vi "target_gm.vi"   [LabVIEW 2011]
uses:
  Input - Cluster gas.ctl
  Output - Cluster gas.ctl
  <vilib>/Platform/TimedLoop/XDataNode/timing_clust.ctl
  <vilib>/Platform/TimedLoop/XDataNode/nitl_modes.ctl
  <vilib>/Platform/TimedLoop/XDataNode/wakeup.ctl
  <vilib>/Platform/TimedLoop/XDataNode/XDataNode.xnode
  <vilib>/Platform/TimedLoop/XDataNode/XDNodeRunTimeDep.lvlib
panel:
  # "The Network Variable Engine and Variable Client Support must be installed on the RT target\nfor this application to function properly. If the Network Variable Engine is not supported on\nthe target (e.g.  FP-2000 with <32MB of RAM), open the project and move the variable library\nto My Computer in the project. Doing this will deploy the variables to localhost but\nwill still require that Variable Client Support be installed on the RT target."
types:
  T1 = typedef "XDNodeRunTimeDep.lvlib/timing_clust.ctl" = cluster{"Expected End [f-1]":u64, "Actual End [f-1]":u64, "Finished Late? [f-1]":bool, "Expected End [i-1]":u64, "Actual End [i-1]":u64, "Finished Late? [i-1]":bool, "Expected Start [i]":u64, "Actual Start [i]":u64, "Expected Start [f]":u64, "Actual Start [f]":u64, "Source Name":string, "Structure Name":string, "Period":i64, "Deadline":i64, "Offset":i64, "Start":i64, "Priority":i32, "Timeout":i32, "Mode":T2, "Wakeup Reason":T3, "Error":errorcluster, "Source Type":string, "Secondary Source Type":string, "Global End Time":u64, "Global Start Time":u64, "Frame Duration":u64, "Iteration Duration":u64, "Assigned CPU":i32, "I/O Scan Engine Mode":u32}
  T2 = typedef "XDNodeRunTimeDep.lvlib/nitl_modes.ctl" = enum32{"No Change", "Process missed periods, maintain original phase", "Discard missed periods, maintain original phase", "Process missed periods, ignore original phase", "Discard missed periods, ignore original phase"}
  T3 = typedef "XDNodeRunTimeDep.lvlib/wakeup.ctl" = enum32{"Normal", "Aborted", "Asynchronous wakeup", "Timing source error", "Timed loop error", "Timeout"}
  T4 = cluster{"STOP":bool, "sqlite_file":string, "gas_values.timestamp":timestamp, "db_write":i64, "output cluster timestamp":timestamp}
  T5 = typedef "Input - Cluster gas.ctl" = cluster{"GM P-1":bool, "GM P-2":bool, "measuring point":u32, "measuring mode":u8, "GM-V1,2":bool, "GM-V3,4":bool, "GM-V5":bool, "measuring volume":u32}
  T6 = typedef "Output - Cluster gas.ctl" = cluster{"B2G2 MR V1.1 AUF":bool, "B2G2 MR V1.1 ZU":bool, "B2G2 MR V1 AUF":bool, "B2G2 MR V1 ZU":bool, "B2G1 T2 V1 AUF":bool, "B2G1 T2 V1 ZU":bool, "B2G1 T2 V1.1 AUF":bool, "B2G1 T2 V1.1 ZU":bool, "B2G2 T2 V1 AUF":bool, "B2G2 T2 V1 ZU":bool, "B2G2 T2 V1.1 ZU":bool, "B2G2 T2 V1.1 AUF":bool, "B2G1 MR V1 AUF":bool, "B2G1 MR V1 ZU":bool, "B2G1 MR V1.1 AUF":bool, "B2G1 MR V1.1 ZU":bool, "B2G1 HR V1 AUF":bool, "B2G1 HR V1 ZU":bool, "B2G1 HR V1.1 AUF":bool, "B2G1 HR V1.1 ZU":bool, "Fab1 HR V1 AUF":bool, "Fab1 HR V1 ZU":bool, "Fab1 HR V1.1 AUF":bool, "Fab1 HR V1.1 ZU":bool, "Fab1 MR V1 AUF":bool, "Fab1 MR V1 ZU":bool, "Fab1 MR V1.1 AUF":bool, "Fab1 MR V1.1 ZU":bool, "Fab1 BL V1 AUF":bool, "Fab1 BL V1 ZU":bool, "Fab1 BL V1.1 AUF":bool, "Fab1 BL V1.1 ZU":bool, "Fab2 HR V1 AUF":bool, "Fab2 HR V1 ZU":bool, "Fab2 HR V1.1 AUF":bool, "Fab2 HR V1.1 ZU":bool, "Fab2 MR V1 AUF":bool, "Fab2 MR V1 ZU":bool, "Fab2 MR V1.1 AUF":bool, "Fab2 MR V1.1 ZU":bool, "GA1 ch4 [%]":dbl, "GA1 co2 [%]":dbl, "GA1 h2 [%]":dbl, "GM P1 RUN":bool, "GM V-1 AUF":bool, "GM V-1 ZU":bool, "GM V-2 AUF":bool, "GM V-2 ZU":bool, "GM V-3 AUF":bool, "GM V-3 ZU":bool, "GM V-4 AUF":bool, "GM V-4 ZU":bool, "GM P2 RUN":bool, "GM GZ-1 [imp]":u32, "GM DS-2 [bar]":dbl, "GM DS-1 [bar]":dbl, "GM TS-1 [°C]":dbl, "GM TS-2[°C]":dbl, "gas_values":cluster{"timestamp":timestamp, "GM DS-2 [bar]":dbl, "GA1 ch4 [%]":dbl, "GA1 co2 [%]":dbl, "GA1 h2 [%]":dbl, "GM DS-1 [bar]":dbl, "GM TS-1 [°C]":dbl, "GM TS-2 [°C]":dbl, "GM GZ-1 [l]":dbl, "empty":bool, "measuring point":u8}, "measuring mode":u8}
  T7 = cluster{"STOP":bool, "measuring point":u32, "measuring mode t-1":u8, "measuring mode t-2":u8, "measuring volume":u32, "gas_values":cluster{"GA1 ch4 [%]":dbl, "GA1 co2 [%]":dbl, "GA1 h2 [%]":dbl, "empty":bool, "measuring point":u8}}
  T8 = cluster{"GA1 ch4 [%]":dbl, "GA1 co2 [%]":dbl, "GA1 h2 [%]":dbl, "empty":bool, "measuring point":u8}
  T9 = cluster{"timestamp":timestamp, "GM DS-2 [bar]":dbl, "GA1 ch4 [%]":dbl, "GA1 co2 [%]":dbl, "GA1 h2 [%]":dbl, "GM DS-1 [bar]":dbl, "GM TS-1 [°C]":dbl, "GM TS-2 [°C]":dbl, "GM GZ-1 [l]":dbl, "empty":bool, "measuring point":u8}
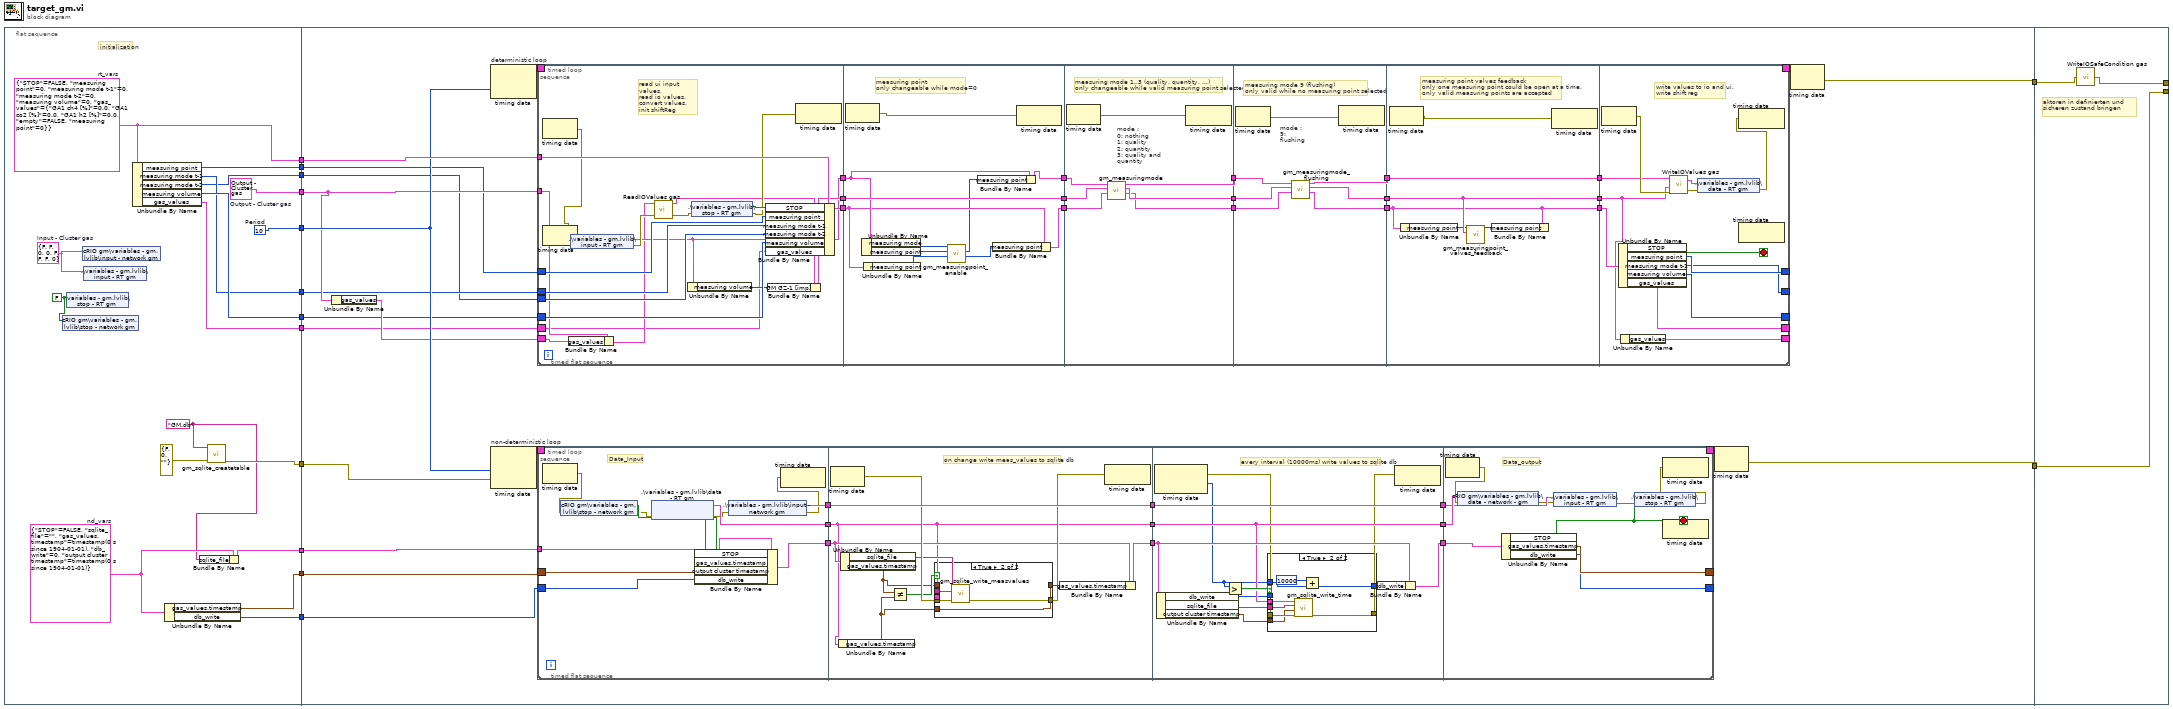
[diagram p0: block diagram]
diagram:
  n1 = flat-sequence {
    tunnel: [w20] -> w14
    tunnel: [w31] -> w13
    tunnel: [w30] -> w12
    tunnel: [w22] -> w9
    tunnel: [w19] -> w8
    tunnel: [w27] -> w7
    tunnel: [w23] -> w6
    tunnel: [w24] -> w5
    tunnel: [w18] -> w4
    tunnel: [w17] -> w3
    tunnel: [w16] -> w2
    tunnel: [w15] -> w1
    tunnel: w14 -> [w46]
    tunnel: w13 -> [w45]
    tunnel: w12 -> [w41]
    tunnel: [w44] -> w11
    tunnel: [w43] -> w10
    tunnel: w9 -> [w42]
    tunnel: w8 -> [w39]
    tunnel: w7 -> [w38]
    tunnel: w6 -> [w37]
    tunnel: w5 -> [w36]
    tunnel: w4 -> [w35]
    tunnel: w3 -> [w34]
    tunnel: w2 -> [w33]
    tunnel: w1 -> [w32]
    tunnel: w11 -> [w304]
    tunnel: w10 -> [w302]
    tunnel: [w303] -> _
    tunnel: [w304] -> _
    frame #0 {
      w26 = FALSE ("stop - RT gas")
      w21 = "GM.db" ("Database File")
      w25 = T4 {"STOP"=FALSE, "sqlite_file"="", "gas_values.timestamp"=timestamp(0 s since 1904-01-01), "db_write"=0, "output cluster timestamp"=timestamp(0 s since 1904-01-01)}  # nd_vars
      w29 = T5 {"GM P-1"=FALSE, "GM P-2"=FALSE, "measuring point"=0, "measuring mode"=0, "GM-V1,2"=FALSE, "GM-V3,4"=FALSE, "GM-V5"=FALSE, "measuring volume"=0}  # Input - Cluster gas
      w30 = T6 {"B2G2 MR V1.1 AUF"=FALSE, "B2G2 MR V1.1 ZU"=FALSE, "B2G2 MR V1 AUF"=FALSE, "B2G2 MR V1 ZU"=FALSE, "B2G1 T2 V1 AUF"=FALSE, "B2G1 T2 V1 ZU"=FALSE, "B2G1 T2 V1.1 AUF"=FALSE, "B2G1 T2 V1.1 ZU"=FALSE, "B2G2 T2 V1 AUF"=FALSE, "B2G2 T2 V1 ZU"=FALSE, "B2G2 T2 V1.1 ZU"=FALSE, "B2G2 T2 V1.1 AUF"=FALSE, "B2G1 MR V1 AUF"=FALSE, "B2G1 MR V1 ZU"=FALSE, "B2G1 MR V1.1 AUF"=FALSE, "B2G1 MR V1.1 ZU"=FALSE, "B2G1 HR V1 AUF"=FALSE, "B2G1 HR V1 ZU"=FALSE, "B2G1 HR V1.1 AUF"=FALSE, "B2G1 HR V1.1 ZU"=FALSE, "Fab1 HR V1 AUF"=FALSE, "Fab1 HR V1 ZU"=FALSE, "Fab1 HR V1.1 AUF"=FALSE, "Fab1 HR V1.1 ZU"=FALSE, "Fab1 MR V1 AUF"=FALSE, "Fab1 MR V1 ZU"=FALSE, "Fab1 MR V1.1 AUF"=FALSE, "Fab1 MR V1.1 ZU"=FALSE, "Fab1 BL V1 AUF"=FALSE, "Fab1 BL V1 ZU"=FALSE, "Fab1 BL V1.1 AUF"=FALSE, "Fab1 BL V1.1 ZU"=FALSE, "Fab2 HR V1 AUF"=FALSE, "Fab2 HR V1 ZU"=FALSE, "Fab2 HR V1.1 AUF"=FALSE, "Fab2 HR V1.1 ZU"=FALSE, "Fab2 MR V1 AUF"=FALSE, "Fab2 MR V1 ZU"=FALSE, "Fab2 MR V1.1 AUF"=FALSE, "Fab2 MR V1.1 ZU"=FALSE, "GA1 ch4 [%]"=0.0, "GA1 co2 [%]"=0.0, "GA1 h2 [%]"=0.0, "GM P1 RUN"=FALSE, "GM V-1 AUF"=FALSE, "GM V-1 ZU"=FALSE, "GM V-2 AUF"=FALSE, "GM V-2 ZU"=FALSE, "GM V-3 AUF"=FALSE, "GM V-3 ZU"=FALSE, "GM V-4 AUF"=FALSE, "GM V-4 ZU"=FALSE, "GM P2 RUN"=FALSE, "GM GZ-1 [imp]"=0, "GM DS-2 [bar]"=0.0, "GM DS-1 [bar]"=0.0, "GM TS-1 [°C]"=0.0, "GM TS-2[°C]"=0.0, "gas_values"={"timestamp"=timestamp(0 s since 1904-01-01), "GM DS-2 [bar]"=0.0, "GA1 ch4 [%]"=0.0, "GA1 co2 [%]"=0.0, "GA1 h2 [%]"=0.0, "GM DS-1 [bar]"=0.0, "GM TS-1 [°C]"=0.0, "GM TS-2 [°C]"=0.0, "GM GZ-1 [l]"=0.0, "empty"=FALSE, "measuring point"=0}, "measuring mode"=0}  # Output - Cluster gas
      w20 = T7 {"STOP"=FALSE, "measuring point"=0, "measuring mode t-1"=0, "measuring mode t-2"=0, "measuring volume"=0, "gas_values"={"GA1 ch4 [%]"=0.0, "GA1 co2 [%]"=0.0, "GA1 h2 [%]"=0.0, "empty"=FALSE, "measuring point"=0}}  # rt_vars
      w31 = i64 10  # Period
      # "initialization"
      n2 = shared-variable "cRIO gm\\variables - gm.lvlib\\stop - network gm"(w26) -> ()  [unwired: 1 in, 1 out]
      n3 = shared-variable ".\\variables - gm.lvlib\\stop - RT gm"(w26) -> ()  [unwired: 1 in, 1 out]
      n4 = shared-variable "cRIO gm\\variables - gm.lvlib\\input - network gm"(w29) -> ()  [unwired: 1 in, 1 out]
      n5 = shared-variable ".\\variables - gm.lvlib\\input - RT gm"(w29) -> ()  [unwired: 1 in, 1 out]
      n6 = Unbundle By Name(w20) -> ("measuring point"=w18:u32, "measuring mode t-1"=w16:u8, "measuring mode t-2"=w15:u8, "measuring volume"=w17:u32, "gas_values"=w19:T8)
      n7 = Unbundle By Name(w25) -> ("gas_values.timestamp"=w23:timestamp, "db_write"=w24:i64)
      n8 = Bundle By Name(cluster=w25, "sqlite_file"=w21) -> (w22:T4)
      n9 = call "gm_sqlite_createtable.vi"("error in (no error)"=errorcluster {"status"=FALSE, "code"=0, "source"=""}, "Database File"=w21) -> ("error out"=w27:errorcluster)  [unwired: 9 in]
    }
    frame #1 {
      n10 = Unbundle By Name(w41) -> ("gas_values"=w40:T9)
      n11 = node-c288 ("Input Node")(w45) -> (w50:T1)  [unwired: 1 in]
      n12 = node-c288 ("Input Node")(w45, w38) -> (w48:T1)  [unwired: 1 in]
      n13 = timed-loop "deterministic loop" {
        timing: w50 -> [_]
        timing-out: [_] -> w49
        tunnel: w46 -> [w173]
        tunnel: w41 -> [w172]
        shift-right: [w171] -> _
        shift-left: w35 -> [w170]
        shift-right: [w169] -> _
        shift-left: w33 -> [w168]
        shift-left: w32 -> [w167]
        shift-right: [w166] -> _
        shift-left: w34 -> [w165]
        shift-right: [w164] -> _
        shift-left: w40 -> [w163]
        shift-right: [w162] -> _
        shift-left: w39 -> [w161]
        stop <- w286 stop-if-true
        n14 = timed-sequence {
          timing: _ -> [_]
          timing-out: _ -> [_]
          tunnel: w173 -> [w201]
          tunnel: w172 -> [w200]
          tunnel: [w193] -> w171
          tunnel: w170 -> [w192]
          tunnel: [w188] -> w169
          tunnel: w168 -> [w187]
          tunnel: w167 -> [w186]
          tunnel: [w185] -> w166
          tunnel: w165 -> [w184]
          tunnel: [w183] -> w164
          tunnel: w163 -> [w182]
          tunnel: [w181] -> w162
          tunnel: w161 -> [w180]
          n15 = timed-flat-sequence {
            tunnel: w201 -> [w220]
            tunnel: w200 -> [w205]
            tunnel: [w207] -> w199
            tunnel: [w216] -> w198
            tunnel: [w208] -> w197
            tunnel: w192 -> [w212]
            tunnel: w187 -> [w211]
            tunnel: w186 -> [w210]
            tunnel: w184 -> [w209]
            tunnel: w182 -> [w203]
            tunnel: w180 -> [w202]
            tunnel: w199 -> [w234]
            tunnel: [w227] -> w191
            tunnel: w198 -> [w231]
            tunnel: [w229] -> w190
            tunnel: w197 -> [w236]
            tunnel: [w236] -> w189
            tunnel: w191 -> [w243]
            tunnel: [w242] -> w179
            tunnel: w190 -> [w245]
            tunnel: [w244] -> w177
            tunnel: w189 -> [w247]
            tunnel: [w246] -> w175
            tunnel: w179 -> [w259]
            tunnel: [w258] -> w178
            tunnel: w177 -> [w255]
            tunnel: [w254] -> w176
            tunnel: w175 -> [w257]
            tunnel: [w256] -> w174
            tunnel: w178 -> [w271]
            tunnel: [w271] -> w196
            tunnel: w176 -> [w266]
            tunnel: [w266] -> w195
            tunnel: w174 -> [w269]
            tunnel: [w269] -> w194
            tunnel: w196 -> [w283]
            tunnel: w195 -> [w287]
            tunnel: w194 -> [w279]
            tunnel: [w282] -> w193
            tunnel: [w281] -> w188
            tunnel: [w280] -> w185
            tunnel: [w278] -> w183
            tunnel: [w277] -> w181
            frame #0 {
              # "read ui input values,\nread io values,\nconvert values,\ninit shiftReg"
              n16 = node-c288 ("Output Node")() -> (w214:errorcluster)  [unwired: 1 in]
              n17 = Bundle By Name(cluster=w205, "gas_values"=w203) -> (w204:T6)
              n18 = shared-variable ".\\variables - gm.lvlib\\input - RT gm"(error in=w214) -> (w207:T5, error out=w213:errorcluster)
              n19 = call "ReadIOValues gas.vi"("error in"=w213, "Output - Cluster gas"=w204) -> ("error out"=w217:errorcluster, "Output - Cluster gas"=w215:T6)  [unwired: 2 in]
              n20 = Unbundle By Name(w207) -> ("measuring volume"=w206:u32)
              n21 = shared-variable ".\\variables - gm.lvlib\\stop - RT gm"(error in=w217) -> (w219:bool, error out=w218:errorcluster)
              n22 = Bundle By Name(cluster=w220, "STOP"=w219, "measuring point"=w212, "measuring mode t-1"=w211, "measuring mode t-2"=w210, "measuring volume"=w209, "gas_values"=w202) -> (w216:T7)
              n23 = Bundle By Name(cluster=w215, "GM GZ-1 [imp]"=w206) -> (w208:T6)
              n24 = node-c288 ("Input Node")(w218) -> ()  [unwired: 1 out]
            }
            frame #1 {
              # "measuring point\nonly changeable while mode=0"
              n25 = node-c288() -> (w235:errorcluster)  [unwired: 1 in]
              n26 = Unbundle By Name(w234) -> ("measuring mode"=w233:u8, "measuring point"=w232:u32)
              n27 = Unbundle By Name(w231) -> ("measuring point"=w230:u32)
              n28 = call "gm_measuringpoint_enable.vi"("shift reg"=w230, "measuring point"=w232, "measuring mode"=w233) -> ("shift reg out"=w228:u32, "measuring point"=w226:u32)  [unwired: 6 in]
              n29 = Bundle By Name(cluster=w234, "measuring point"=w226) -> (w227:T5)
              n30 = Bundle By Name(cluster=w231, "measuring point"=w228) -> (w229:T7)
              n31 = node-c288(w235) -> ()  [unwired: 1 out]
            }
            frame #2 {
              # "measuring mode 1..3 (quality, quantity, ...)\nonly changeable while valid measuring point selected"
              # "mode :\n0: nothing\n1: quality\n2: quantity\n3: quality and quantity"
              n32 = node-c288() -> (w248:errorcluster)  [unwired: 1 in]
              n33 = call "gm_measuringmode.vi"("rt_vars in"=w245, "Output - Cluster gas in"=w247, "Input - Cluster gas in"=w243) -> ("rt_vars out"=w244:T7, "Output - Cluster gas out"=w246:T6, "Input - Cluster gas out"=w242:T5)  [unwired: 6 in]
              n34 = node-c288(w248) -> ()  [unwired: 1 out]
            }
            frame #3 {
              # "mode :\n9: flushing"
              # "measuring mode 9 (flushing)\nonly valid while no measuring point selected"
              n35 = node-c288() -> (w260:errorcluster)  [unwired: 1 in]
              n36 = call "gm_measuringmode_flushing.vi"("rt_vars in"=w255, "Output - Cluster gas in"=w257, "Input - Cluster gas in"=w259) -> ("rt_vars out"=w254:T7, "Output - Cluster gas out"=w256:T6, "Input - Cluster gas out"=w258:T5)  [unwired: 6 in]
              n37 = node-c288(w260) -> ()  [unwired: 1 out]
            }
            frame #4 {
              # "measuring point valves feedback \nonly one measuring point could be open at a time,\nonly valid measuring points are accepted"
              n38 = node-c288() -> (w270:errorcluster)  [unwired: 1 in]
              n39 = Unbundle By Name(w266) -> ("measuring point"=w268:u32)
              n40 = call "gm_measuringpoint_valves_feedback.vi"("Output - Cluster gas"=w269, "measuring point"=w268) -> ("measuring point"=w267:u32)  [unwired: 9 in]
              n41 = Bundle By Name(cluster=w266, "measuring point"=w267) -> ()  [unwired: 1 out]
              n42 = node-c288(w270) -> ()  [unwired: 1 out]
            }
            frame #5 {
              # "write values to io and ui,\nwrite shift reg"
              n43 = node-c288() -> (w285:errorcluster)  [unwired: 1 in]
              n44 = Unbundle By Name(w287) -> ("STOP"=w286:bool, "measuring point"=w282:u32, "measuring mode t-1"=w281:u8, "measuring volume"=w280:u32, "gas_values"=w277:T8)
              n45 = Unbundle By Name(w279) -> ("gas_values"=w278:T9)
              n46 = call "WriteIOValues gas.vi"("error in"=w285, "Output - Cluster gas"=w279, "input cluster"=w283) -> ("error out"=w284:errorcluster, "Output - Cluster gas 2"=w289:T6)  [unwired: 1 in]
              n47 = shared-variable ".\\variables - gm.lvlib\\data - RT gm"(w289, error in=w284) -> (error out=w288:errorcluster)
              n48 = node-c288(w288) -> ()  [unwired: 1 out]
            }
          }
        }
        n49 = node-c288() -> ()  [unwired: 1 in, 1 out]
        n50 = node-c288() -> ()  [unwired: 1 in, 1 out]
      }
      n51 = timed-loop "non-deterministic loop" {
        timing: w48 -> [_]
        timing-out: [_] -> w47
        tunnel: w42 -> [w55]
        shift-right: [w54] -> _
        shift-left: w37 -> [w53]
        shift-right: [w52] -> _
        shift-left: w36 -> [w51]
        stop <- w144 stop-if-true
        n52 = timed-sequence {
          timing: _ -> [_]
          timing-out: _ -> [_]
          tunnel: w55 -> [w69]
          tunnel: [w68] -> w54
          tunnel: w53 -> [w67]
          tunnel: [w60] -> w52
          tunnel: w51 -> [w56]
          n53 = timed-flat-sequence {
            tunnel: [w78] -> w58
            tunnel: [w79] -> w59
            tunnel: w69 -> [w81]
            tunnel: [w80] -> w57
            tunnel: w67 -> [w72]
            tunnel: w56 -> [w70]
            tunnel: w59 -> [w97]
            tunnel: [w97] -> w66
            tunnel: w58 -> [w92]
            tunnel: [w92] -> w64
            tunnel: w57 -> [w94]
            tunnel: [w91] -> w62
            tunnel: w66 -> [w121]
            tunnel: [w121] -> w65
            tunnel: w64 -> [w116]
            tunnel: [w116] -> w63
            tunnel: w62 -> [w120]
            tunnel: [w119] -> w61
            tunnel: w65 -> [w145]
            tunnel: w63 -> [w146]
            tunnel: w61 -> [w147]
            tunnel: [w139] -> w68
            tunnel: [w138] -> w60
            frame #0 {
              # "Data_Input"
              n54 = node-c288() -> (w76:errorcluster)  [unwired: 1 in]
              n55 = shared-variable "cRIO gm\\variables - gm.lvlib\\stop - network gm"(error in=w76) -> (w77:bool, error out=w75:errorcluster)
              n56 = shared-variable ".\\variables - gm.lvlib\\data - RT gm"(error in=w75) -> (w78:T6, error out=w74:errorcluster, w71:timestamp)
              n57 = Bundle By Name(cluster=w81, "STOP"=w77, "gas_values.timestamp"=w72, "output cluster timestamp"=w71, "db_write"=w70) -> (w80:T4)
              n58 = shared-variable ".\\variables - gm.lvlib\\input - network gm"(error in=w74) -> (w79:T5, error out=w73:errorcluster)
              n59 = node-c288(w73) -> ()  [unwired: 1 out]
            }
            frame #1 {
              # "on change write meas_values to sqlite db"
              n60 = node-c288() -> (w96:errorcluster)  [unwired: 1 in]
              n61 = Unbundle By Name(w92) -> ("gas_values.timestamp"=w87:timestamp)
              n62 = Unbundle By Name(w94) -> ("sqlite_file"=w93:string, "gas_values.timestamp"=w88:timestamp)
              n63 = Not Equal?(x=w88, y=w87) -> (x != y?=w90:bool)
              n64 = case shown="True" w90 {
                tunnel: w96 -> [w98 w104]
                tunnel: [w98 w103] -> w95
                tunnel: w93 -> [_ w102]
                tunnel: w92 -> [_ w101]
                tunnel: [w99 w100] -> w89
                tunnel: w88 -> [w99 _]
                tunnel: w87 -> [_ w100]
                frame False {
                }
                frame True {
                  n65 = call "gm_sqlite_write_measvalues.vi"("error in (no error)"=w104, "Database File"=w102, "Output - Cluster gas"=w101) -> ("error out"=w103:errorcluster)  [unwired: 8 in]
                }
              }
              n66 = Bundle By Name(cluster=w94, "gas_values.timestamp"=w89) -> (w91:T4)
              n67 = node-c288(w95) -> ()  [unwired: 1 out]
            }
            frame #2 {
              # "every interval (10000ms) write values to sqlite db"
              n68 = node-c288() -> (w115:errorcluster, w111:i64)  [unwired: 1 in]
              n69 = Unbundle By Name(w120) -> ("db_write"=w110:i64, "sqlite_file"=w113:string, "output cluster timestamp"=w112:timestamp)
              n70 = Greater?(x=w111, y=w110) -> (0:w117:bool)
              n71 = case shown="True" w117 {
                tunnel: w111 -> [_ w131]
                tunnel: w110 -> [w123 _]
                tunnel: [w123 w130] -> w118
                tunnel: w116 -> [_ w128]
                tunnel: w115 -> [w122 w127]
                tunnel: [w122 w126] -> w114
                tunnel: w113 -> [_ w125]
                tunnel: w112 -> [_ w124]
                frame False {
                }
                frame True {
                  n72 = call "gm_sqlite_write_time.vi"("error in (no error)"=w127, "output cluster timestamp"=w124, "Database File"=w125, "Output - Cluster gas"=w128) -> ("error out"=w126:errorcluster)  [unwired: 7 in]
                  n73 = Add(x=i64 10000, y=w131) -> (x+y=w130:i64)
                }
              }
              n74 = Bundle By Name(cluster=w120, "db_write"=w118) -> (w119:T4)
              n75 = node-c288(w114) -> ()  [unwired: 1 out]
            }
            frame #3 {
              # "Data_output"
              n76 = node-c288() -> (w143:errorcluster)  [unwired: 1 in]
              n77 = shared-variable "cRIO gm\\variables - gm.lvlib\\data - network - gm"(w146, error in=w143) -> (error out=w142:errorcluster)
              n78 = Unbundle By Name(w147) -> ("STOP"=w144:bool, "gas_values.timestamp"=w139:timestamp, "db_write"=w138:i64)
              n79 = shared-variable ".\\variables - gm.lvlib\\input - RT gm"(w145, error in=w142) -> (error out=w141:errorcluster)
              n80 = shared-variable ".\\variables - gm.lvlib\\stop - RT gm"(w144, error in=w141) -> (error out=w140:errorcluster)
              n81 = node-c288(w140) -> ()  [unwired: 1 out]
            }
          }
        }
        n82 = node-c288() -> ()  [unwired: 1 in, 1 out]
        n83 = node-c288() -> ()  [unwired: 1 in, 1 out]
      }
      n84 = node-c288 ("Output Node")(w47) -> (w44:errorcluster)
      n85 = node-c288 ("Output Node")(w49) -> (w43:errorcluster)
    }
    frame #2 {
      # "aktoren in definierten und sicheren zustand bringen"
      n86 = call "WriteIOSafeCondition gas.vi"("error in"=w302) -> ("error out"=w303:errorcluster)
    }
  }
